vi "RefreshEntireTree.vi"(7 "calling VI in":refnum<vi>, 8 "error in":errorcluster, 10 "array":T1[](array[typedef]), 11 "tree ref in":refnum<vi>) -> (0 "error out":errorcluster)   [LabVIEW 2013, in "NISE_CEF_TreeControl.lvlib"]
doc: "This VI refreshes the complete tree based on the node summary"
uses:
  NISE_CEF_TreeControl.lvlib
  Node/Summary.ctl
  Node/NISE_CEF_Node.lvclass
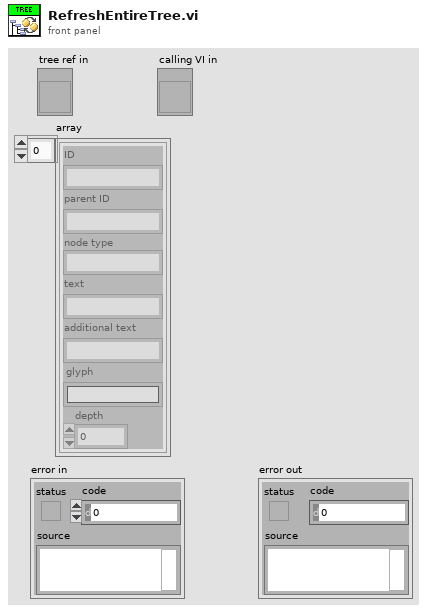
[diagram p1: front panel]
types:
  T1 = typedef "NISE_CEF_Node.lvclass/Summary.ctl" = cluster{"ID":string, "parent ID":string, "node type":string, "text":string, "additional text":string, "glyph":string, "depth":i32}
  T2 = cluster{"Left Cell String":string, "Child text":string[], "Child Tag":string, "Item Indent":i32, "Child Only?":bool, "glyph Index":i32}
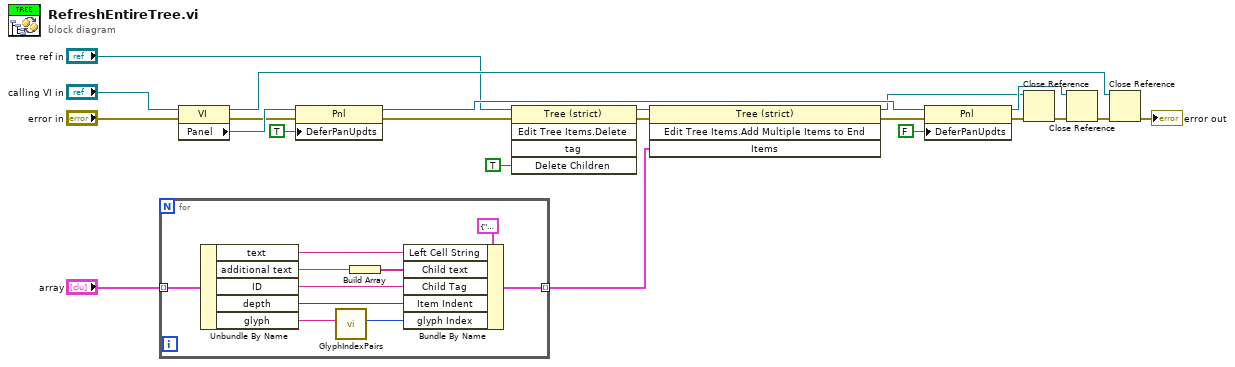
[diagram p0: block diagram]
diagram:
  n1 = for {
    tunnel: "array" -> [w32] mode=indexing
    tunnel: [w30] -> w3 mode=indexing
    n2 = Unbundle By Name(w32) -> ("text"=w29:string, "additional text"=w27:string, "ID"=w26:string, "depth"=w25:i32, "glyph"=w24:string)
    n3 = call "GlyphIndexPairs.vi"("glyph"=w24) -> ("index"=w23:i32)  [unwired: 10 in]
    n4 = Build Array(w27) -> (w28:string[])
    n5 = Bundle By Name(cluster=T2 {"Left Cell String"="", "Child text"=[], "Child Tag"="", "Item Indent"=0, "Child Only?"=FALSE, "glyph Index"=0} ("Item"), "Left Cell String"=w29, "Child text"=w28, "Child Tag"=w26, "Item Indent"=w25, "glyph Index"=w23) -> (w30:T2)
  }
  n6 = property class="VI"(reference="calling VI in", error in="error in") -> (reference out=w12:refnum<vi>, error out=w20:errorcluster, "Panel"=w21:refnum<vi>)
  n7 = property class="Pnl"(reference=w21, error in=w20, "DeferPanUpdts"=TRUE ("Defer Panel Updates")) -> (reference out=w16:refnum<vi>, error out=w4:errorcluster)
  n8 = invoke class="Tree (strict)" method="Edit Tree Items.Delete"(reference="tree ref in", error in=w4, "Delete Children"=TRUE ("Delete Children?")) -> (reference out=w6:refnum<vi>, error out=w2:errorcluster)  [unwired: 2 in, 3 out]
  n9 = invoke class="Tree (strict)" method="Edit Tree Items.Add Multiple Items to End"(reference=w6, error in=w2, "Items"=w3) -> (reference out=w5:refnum<vi>, error out=w1:errorcluster)  [unwired: 1 in, 2 out]
  n10 = property class="Pnl"(reference=w16, error in=w1, "DeferPanUpdts"=FALSE ("Defer Panel Updates")) -> (reference out=w13:refnum<vi>, error out=w15:errorcluster)
  n11 = Close Reference(reference=w5, error in (no error)=w15) -> (error out=w14:errorcluster)
  n12 = Close Reference(reference=w13, error in (no error)=w14) -> (error out=w11:errorcluster)
  n13 = Close Reference(reference=w12, error in (no error)=w11) -> (error out=→"error out":errorcluster)
